vi "AttackerPenalty.vi"(4 "AI Parameters":T8={"GotoKick"={"Dist do cone a frente"=150.0, "attacker farback"=1500.0, "Perto"=300.0, "min dist to kick"=150.0, "kick eps"=0.0, "Time to transition"=0.05}, "Attacker"={"CC chute"=0.09, "CC passe"=0.045, "Kick Force"=100.0, "ball-robot Kick"=200.0, "ball-robot Pass"=0.3, "drible\nAttk"=FALSE}, "Defender"={"D max"=1700.0, "Vel p/ robô av"=1000.0, "Kick Force"=100.0, "D atk-def"=0.0, "D farback"=0.0, "drible\ndef"=FALSE, "drible\ngoalie"=FALSE}, "Timeout"={"Field/v in x"=6.0, "Dist Robots"=300, "Dist up in y"=300}, "Pose Striker"={"dist"=200.0, "Numeric"=-4.0, "dist 2"=200.0, "drible\nstriker"=FALSE}, "Dist Stop"=300.0, "D ball out"=200, "D central gap "=150.0, "T pass"=0.0, "Force ++"=0.0, "range kick"=0.0, "Chute alto"=TRUE, "Marcador novo"=TRUE, "drible"=FALSE, "D drible"=300.0, "Versão Striker"=enum."Auto", "Defesa"=enum."ManMark", "Marcador"=enum."Marcar Segundo mais perigoso", "Receptor passe"=enum."Auto", "Área"=enum."Quadrada", "Decisão\nsimples?"=FALSE} {"D drible" format="%#_13g"; "D central gap" format="%#_13g"; "Dist Stop" format="%#_13g"; "Pose Striker"."Numeric" format="%#_13g"; "Defender"."Kick Force" format="%#_13g"; "Defender"."Vel p/ robô av" format="%#_13g"; "Attacker"."ball-robot Kick" format="%#_13g"; "Attacker"."Kick Force" format="%#_13g"; "Attacker"."CC passe" format="%#_13g"; "Attacker"."CC chute" format="%#_13g"; "GotoKick"."kick eps" format="%#_13g"; "GotoKick"."min dist to kick" format="%#_13g"; "GotoKick"."Perto" format="%#_13g"; "GotoKick"."attacker farback" format="%#_13g"; "GotoKick"."Dist do cone a frente" format="%#_13g"}, 7 "IA State Input":T9={"our_robots"=[], "enemy_robots"=[], "balls"=[], "geometry"={"line_width"=0, "field_length"=0, "field_width"=0, "boundary_width"=0, "referee_width"=0, "goal_width"=0, "goal_depth"=0, "goal_wall_width"=0, "center_circle_radius"=0, "defense_radius"=0, "defense_stretch"=0, "free_kick_from_defense_dist"=0, "penalty_spot_from_field_line_dist"=0, "penalty_line_from_spot_dist"=0}, "IA Judge"={"stage"="", "command"="", "our_goalie_id"=0.0, "enemy_goalie_id"=0.0, "command enum"=enum."Halt", "Time"=enum."Azul"}, "Received Timestamp"=timestamp(0 s since 1904-01-01), "Events"={"Touch"=FALSE, "Ball out"=FALSE, "id touch"=0.0, "Ball out of \nVision"=FALSE, "Ball inside \nGoalie area"=FALSE, "Robot not responding"=FALSE, "Robots responding status"=[1.0, 1.0, 1.0, 1.0, 1.0, 1.0], "Enemy Ball \nPossession"=FALSE, "Pass State"=FALSE, "id end of pass"=0.0, "Kick"=FALSE, "Id ini Possession"=0.0, "Ball Possesion"=FALSE, "Id Possesion"=0.0, "Direct Kick"=FALSE, "2nd Strk Ativo"=FALSE}}, 8 "atacando contra?":bool=TRUE, 9 "balls":T6[](array[typedef]), 10 "geometry":T7, 11 "Robot in":T1={"id"=0, "function"=enum."Attacker", "x"=0.0, "y"=0.0, "orientation"=0.0, "v_tangent"=0.0, "v_normal"=0.0, "v_ang"=0.0, "kick_x"=0.0, "kick_z"=0.0, "dribble"=FALSE, "Timestamp"=timestamp(0 s since 1904-01-01), "estimatives"={"est_v_tangent"=0.0, "est_v_normal"=0.0, "est_vx"=0.0, "est_vy"=0.0, "Pos Robot Est"=[]}, "dest_x_kick"=0.0, "dest_y_kick"=0.0, "Gap Coord"=[], "States"=enum."GoToTangent", "Path "=[], "Path  Smooth"=[], "Dest"=[]}) -> (2 "Robot out":T1={"id"=5, "function"=enum."Attacker", "x"=-1842.5054931640625, "y"=520.60986328125, "orientation"=-2.7555055618286133, "v_tangent"=-0.08361641967936218, "v_normal"=-0.20513016702014014, "v_ang"=0.24456003022714357, "kick_x"=0.0, "kick_z"=0.0, "dribble"=FALSE, "Timestamp"=timestamp(2082758857.4639893 s since 1904-01-01), "estimatives"={"est_v_tangent"=0.0, "est_v_normal"=0.0, "est_vx"=0.0, "est_vy"=0.0, "Pos Robot Est"=[]}, "dest_x_kick"=0.0, "dest_y_kick"=0.0, "Gap Coord"=[], "States"=enum."GoToTangent", "Path "=[], "Path  Smooth"=[], "Dest"=[]})   [LabVIEW 2018]
uses:
  Core/AI Input.ctl
  Core/AI Robot.ctl
  Functions Enum.ctl
  AttackerStates.ctl
  Path Planning/RRT/PathDests.ctl
  Path Planning/RRT/PathDest.ctl
  Core/AI Ball.ctl
  Core/Field Size.ctl
  Core/AI Judge.ctl
  Command Enum.ctl
  Util/Events/Events.ctl
  AI Parameters.ctl
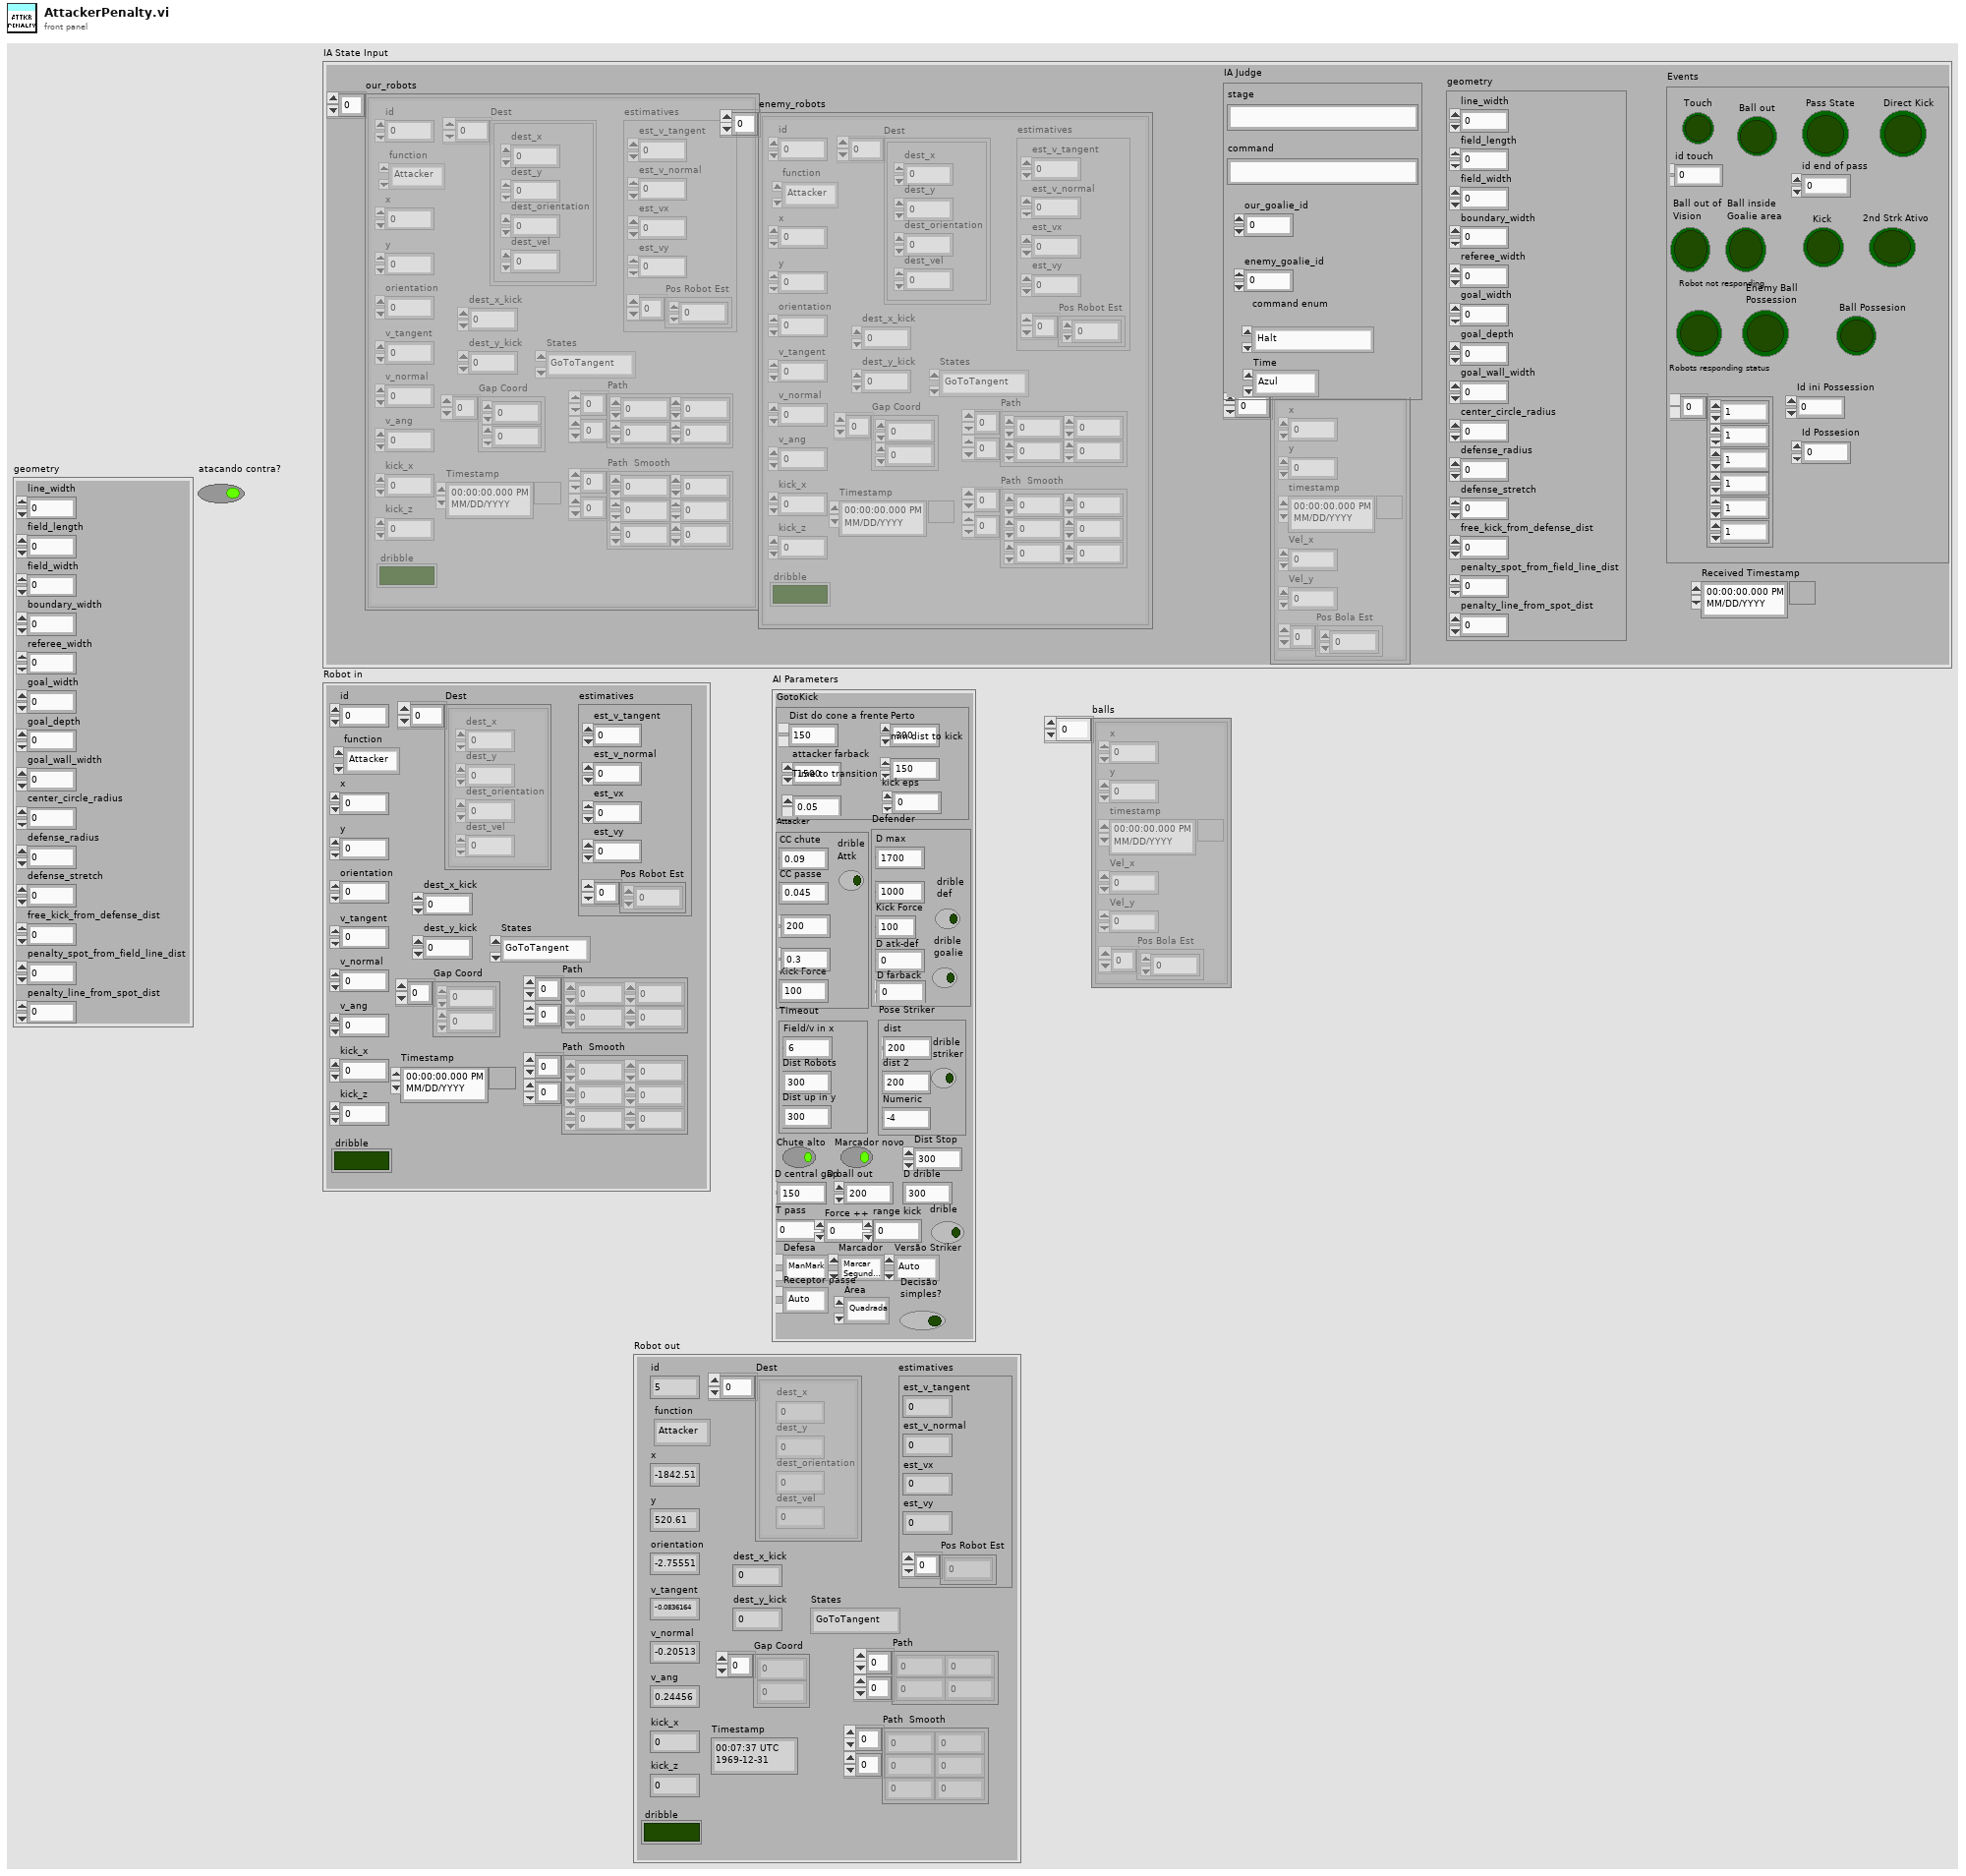
[diagram p1: front panel]
types:
  T1 = typedef "AI Robot.ctl" = cluster{"id":u32, "function":T2, "x":dbl, "y":dbl, "orientation":dbl, "v_tangent":dbl, "v_normal":dbl, "v_ang":dbl, "kick_x":dbl, "kick_z":dbl, "dribble":bool, "Timestamp":timestamp, "estimatives":cluster{"est_v_tangent":dbl, "est_v_normal":dbl, "est_vx":dbl, "est_vy":dbl, "Pos Robot Est":dbl[]}, "dest_x_kick":dbl, "dest_y_kick":dbl, "Gap Coord":dbl[], "States":T3, "Path ":dbl[][], "Path  Smooth":dbl[][], "Dest":T4}
  T2 = typedef "Functions Enum.ctl" = enum16{"2nd Striker", "Attacker", "Goalie", "Defender", "Striker", "Goto 0", "Dummy", "Kicker", "ZigZag 0", "ZigZag 1", "ZigZag 2", "ZigZag 3", "ZigZag 4", "ZigZag 5", "ZigZag 6", "ZigZag 7", "ZigZag 8", ""}
  T3 = typedef "AttackerStates.ctl" = enum16{"Pass", "GoToTangent", "BallGetting", "GoToKick", ""}
  T4 = typedef "PathDests.ctl" = T5[]
  T5 = typedef "PathDest.ctl" = cluster{"dest_x":dbl, "dest_y":dbl, "dest_orientation":dbl, "dest_vel":dbl}
  T6 = typedef "AI Ball.ctl" = cluster{"x":dbl, "y":dbl, "timestamp":timestamp, "Vel_x":dbl, "Vel_y":dbl, "Pos Bola Est":dbl[]}
  T7 = typedef "Field Size.ctl" = cluster{"line_width":u32, "field_length":u32, "field_width":u32, "boundary_width":u32, "referee_width":u32, "goal_width":u32, "goal_depth":u32, "goal_wall_width":u32, "center_circle_radius":u32, "defense_radius":u32, "defense_stretch":u32, "free_kick_from_defense_dist":u32, "penalty_spot_from_field_line_dist":u32, "penalty_line_from_spot_dist":u32}
  T8 = typedef "AI Parameters.ctl" = cluster{"GotoKick":cluster{"Dist do cone a frente":dbl, "attacker farback":dbl, "Perto":dbl, "min dist to kick":dbl, "kick eps":dbl, "Time to transition":dbl}, "Attacker":cluster{"CC chute":dbl, "CC passe":dbl, "Kick Force":dbl, "ball-robot Kick":dbl, "ball-robot Pass":dbl, "drible\nAttk":bool}, "Defender":cluster{"D max":dbl, "Vel p/ robô av":dbl, "Kick Force":dbl, "D atk-def":dbl, "D farback":dbl, "drible\ndef":bool, "drible\ngoalie":bool}, "Timeout":cluster{"Field/v in x":dbl, "Dist Robots":u32, "Dist up in y":u32}, "Pose Striker":cluster{"dist":dbl, "Numeric":dbl, "dist 2":dbl, "drible\nstriker":bool}, "Dist Stop":dbl, "D ball out":i32, "D central gap ":dbl, "T pass":dbl, "Force ++":dbl, "range kick":dbl, "Chute alto":bool, "Marcador novo":bool, "drible":bool, "D drible":dbl, "Versão Striker":enum16{"Auto", "3", "2", "1"}, "Defesa":enum16{"ManMark", "Barreira"}, "Marcador":enum16{"Marcar Segundo mais perigoso", "Marcar o mais perigoso"}, "Receptor passe":enum16{"Auto", "2nd Striker", "Striker"}, "Área":enum16{"Quadrada", "Circular"}, "Decisão\nsimples?":bool}
  T9 = typedef "AI Input.ctl" = cluster{"our_robots":T1[], "enemy_robots":T1[], "balls":T6[], "geometry":T7, "IA Judge":T10, "Received Timestamp":timestamp, "Events":T12}
  T10 = typedef "AI Judge.ctl" = cluster{"stage":string, "command":string, "our_goalie_id":dbl, "enemy_goalie_id":dbl, "command enum":T11, "Time":enum16{"Azul", "Amarelo"}}
  T11 = typedef "Command Enum.ctl" = enum16{"Halt", "Stop", "Force Start", "PKA Normal Start", "Prepare Kickoff Ally", "PKE Normal Start", "Prepare Kickoff Enemy", "Prepare Penalty Ally", "PPA Normal Start", "Prepare Penalty Enemy", "PPE Normal Start", "Direct Free Enemy", "Direct Free Ally", "Indirect Free Enemy", "Indirect Free Ally", "Timeout Enemy", "Timeout Ally", "Goal Enemy", "Goal Ally", "Ball Placement Enemy", "Ball Placement Ally", "Normal Half Time", "Extra Time Break", "Extra Half Time", "None", "Post Game"}
  T12 = typedef "Events.ctl" = cluster{"Touch":bool, "Ball out":bool, "id touch":dbl, "Ball out of \nVision":bool, "Ball inside \nGoalie area":bool, "Robot not responding":bool, "Robots responding status":dbl[], "Enemy Ball \nPossession":bool, "Pass State":bool, "id end of pass":dbl, "Kick":bool, "Id ini Possession":dbl, "Ball Possesion":bool, "Id Possesion":dbl, "Direct Kick":bool, "2nd Strk Ativo":bool}
  T13 = cluster{"CC chute":dbl, "CC passe":dbl, "Kick Force":dbl, "ball-robot Kick":dbl, "ball-robot Pass":dbl, "drible\nAttk":bool}
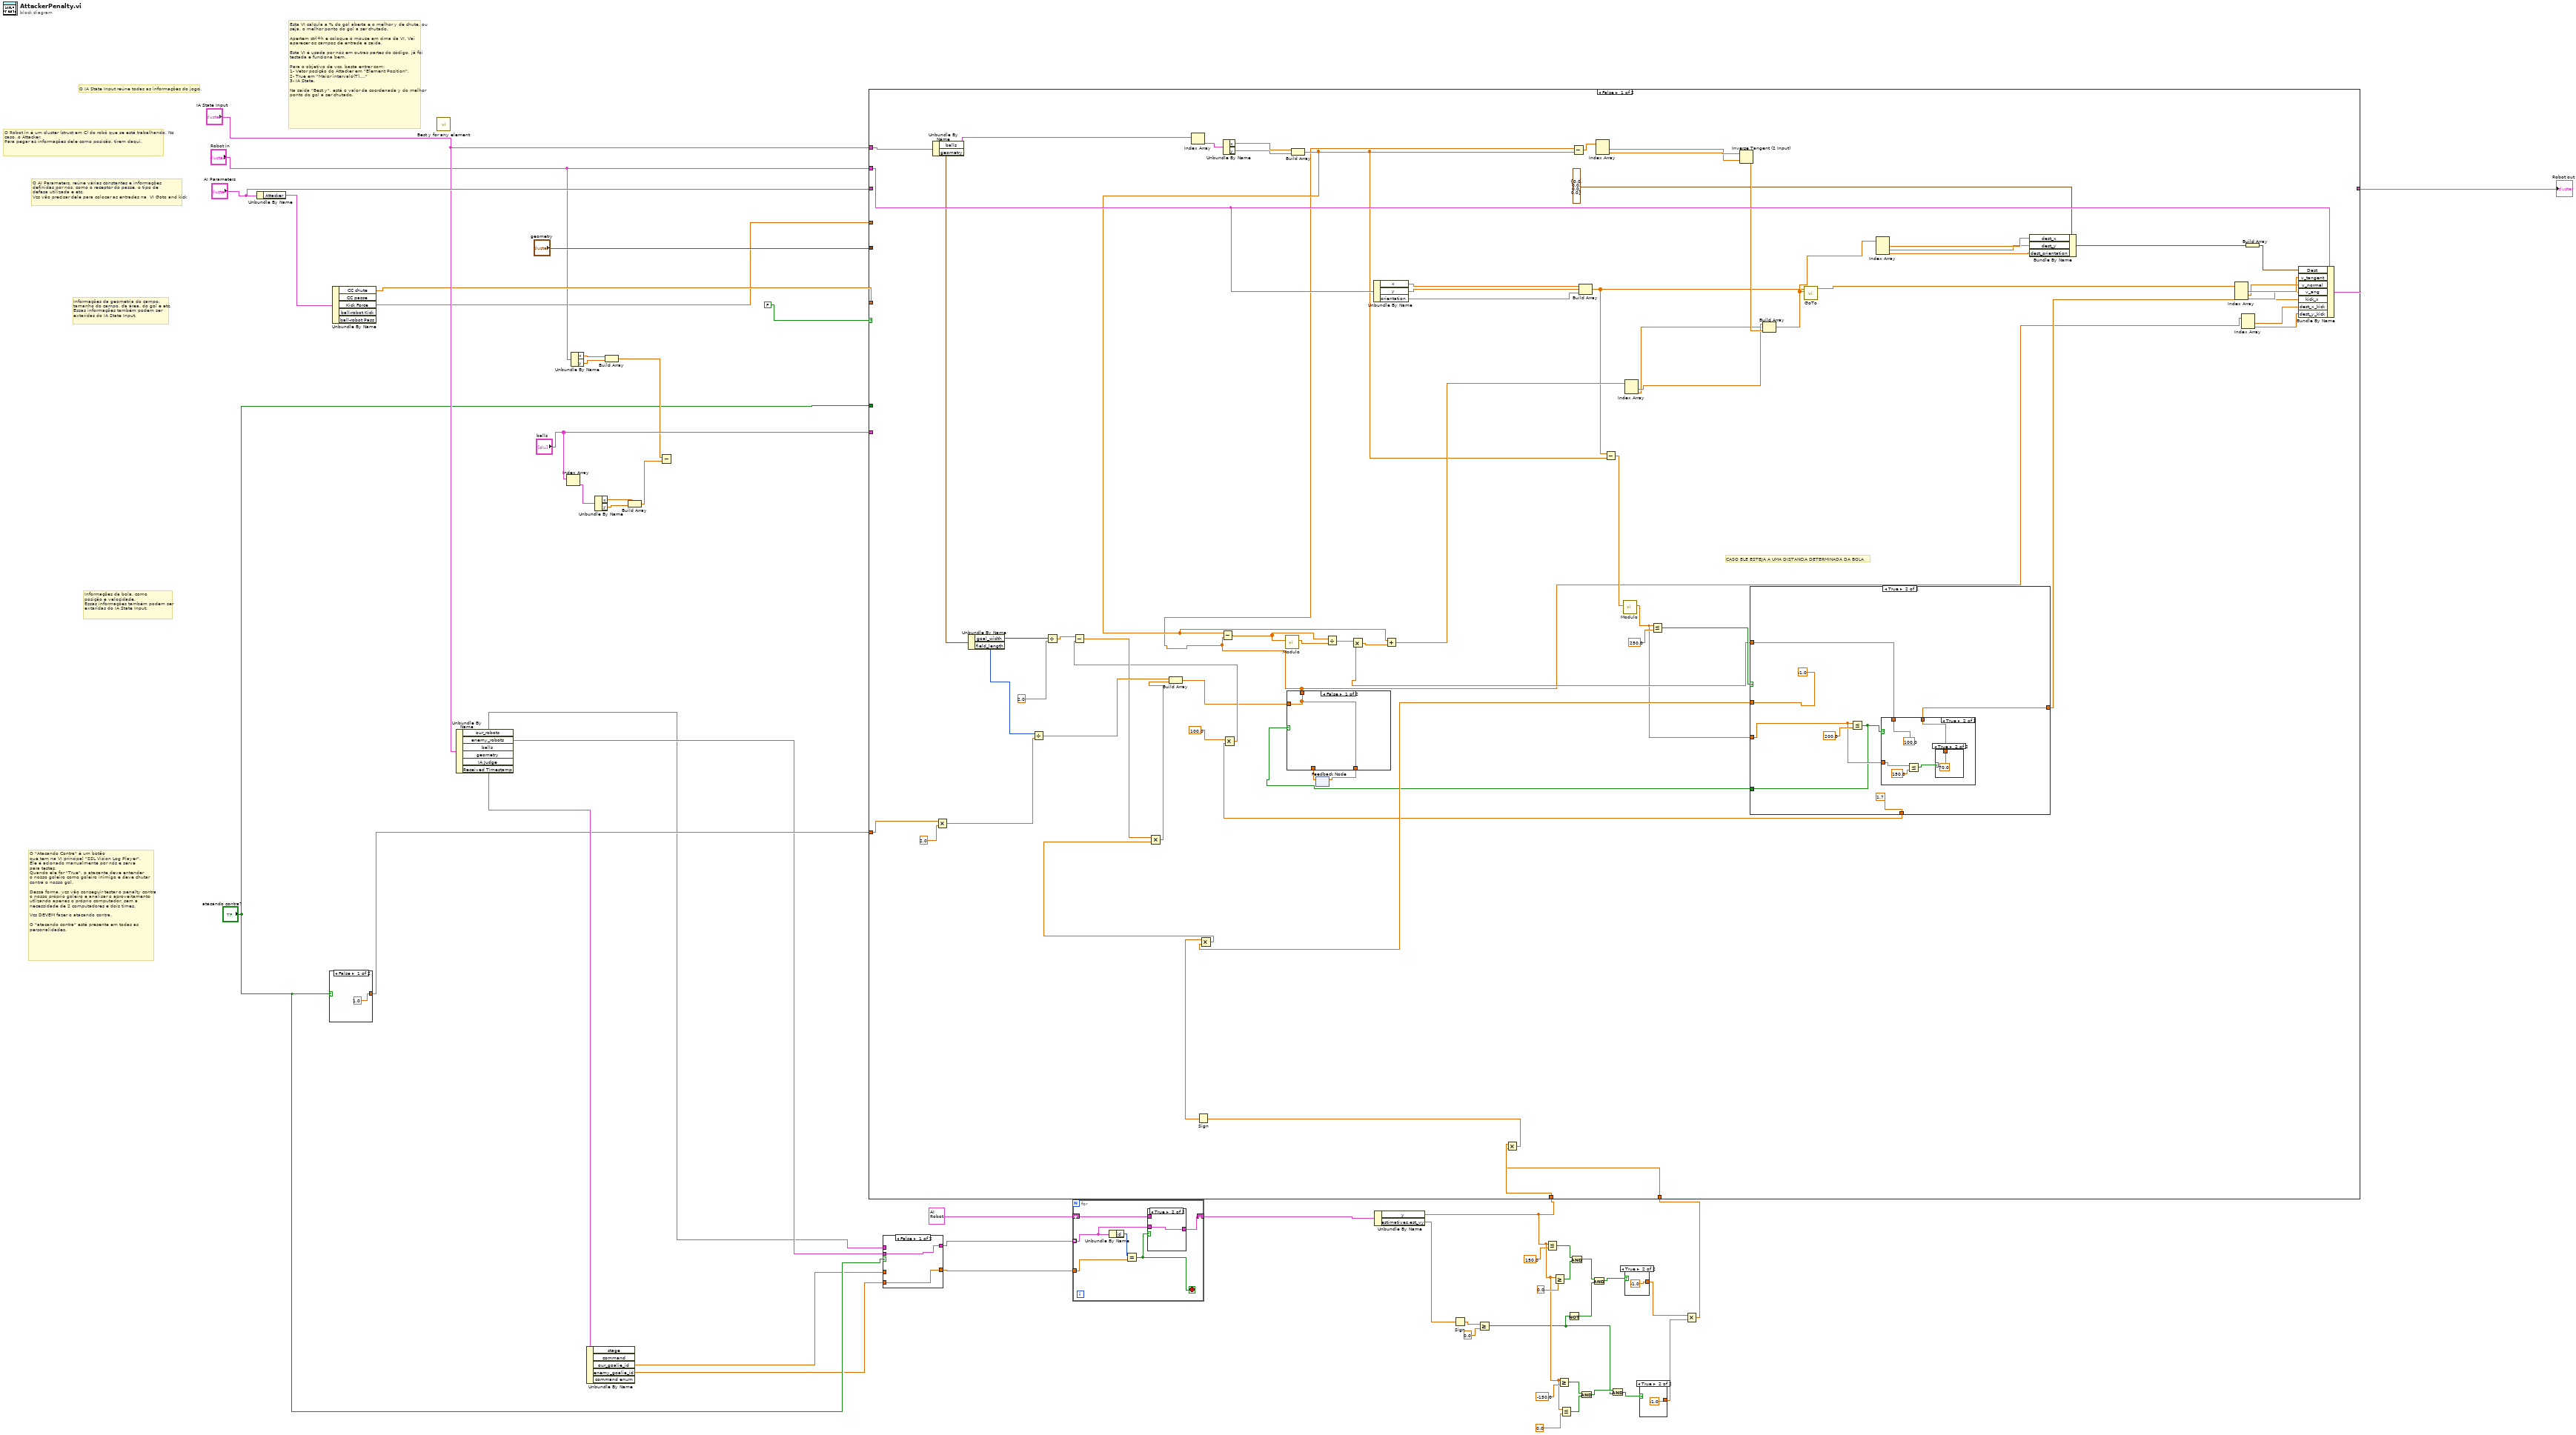
[diagram p0: block diagram]
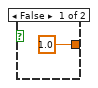
[diagram p2: hidden frame]
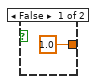
[diagram p3: hidden frame]
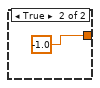
[diagram p5: hidden frame]
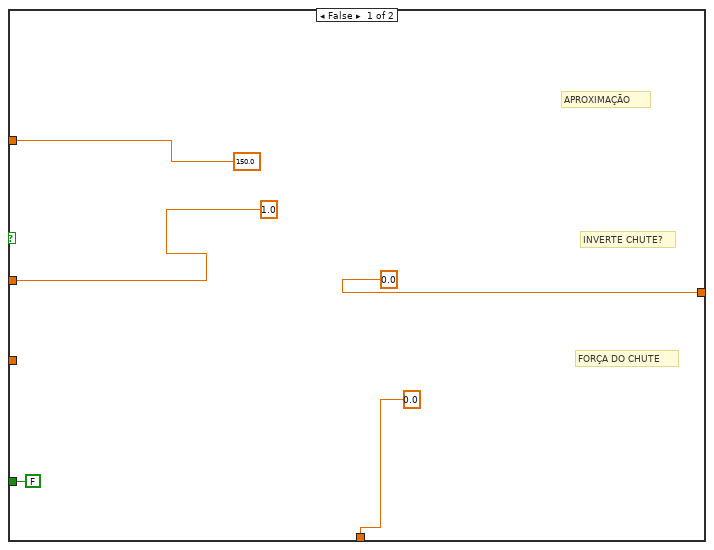
[diagram p8: hidden frame]
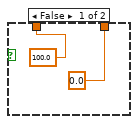
[diagram p9: hidden frame]
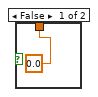
[diagram p10: hidden frame]
diagram:
  # "O \"Atacando Contra\" é um botão\nque tem na VI principal \"SSL Vision Log Player\".\nEle é acionado manualmente por nós e serve\npara testes.\nQuando ele for \"True\", o atacante deve entender \no nosso goleiro como goleiro inimigo e deve chutar\ncontra o nosso gol.\n\nDessa forma, vcs vão conseguir testar o penalty contra\no nosso próprio goleiro e analisar o aproveitamento\nutlizando apenas o próprio computador, sem a\nnecessidade de 2 computadores e dois times.\n\nVcs DEVEM fazer o atacando contra. \n\nO \"atacando contra\" está presente em todas as\npersonalidades."
  # "Informações da bola, como\nposição e velocidade.\nEssas informações também podem ser\nextarídas do IA State Input."
  # "Informações da geometria do campo.\ntamanho do campo, da área, do gol e etc.\nEssas informações também podem ser\nextarídas do IA State Input."
  # "O AI Parameters, reúne várias constantes e informações\ndefinidas por nós, como o receptor do passe, o tipo de\ndefesa utilizada e etc.\nVcs vão precisar dele para colocar as entradas na  VI Goto and kick"
  # "O Robot in é um cluster (struct em C) do robô que se está trabalhando. No caso, o Attacker.\nPara pegar as informações dele como posicão, tirem daqui."
  # "O IA State Input reúne todas as informações do jogo."
  # "Esta VI calcula a % do gol aberta e o melhor y de chute, ou seja, o melhor ponto do gol a ser chutado.\n\nApertem ctrl+h e coloque o mouse em cima da VI. Vai aparecer os campos de entrada e saída.\n\nEsta VI é usada por nós em outras partes do código, já foi testada e funciona bem.\n\nPara o objetivo de vcs, basta entrar com:\n1- Vetor posição do Attacker em \"Element Position\".\n2- True em \"Maior intervalo(T)....\"\n3- IA State.\n\nNa saída \"Best y\", está o valor da coordenada y do melhor ponto do gol a ser chutado."
  n1 = Unbundle By Name("AI Parameters") -> ("Attacker"=w49:T13)
  n2 = case shown="False" "atacando contra?" {
    tunnel: [1.0 -1.0] -> w44
    frame False {
    }
    frame True {
    }
  }
  n3 = Unbundle By Name(w49) -> ("CC chute"=w42:dbl, "Kick Force"=w23:dbl)  [unwired: 3 out]
  n4 = call "Best y for any element.vi"() -> ()  [unwired: 7 in, 5 out]
  n5 = Unbundle By Name("IA State Input") -> ("our_robots"=w25:T1[], "enemy_robots"=w29:T1[], "IA Judge"=w45:T10)  [unwired: 3 out]
  n6 = Index Array(array="balls") -> (element=w39:T6)  [unwired: 1 in]
  n7 = Unbundle By Name("Robot in") -> ("x"=w36:dbl, "y"=w35:dbl)
  n8 = Unbundle By Name(w45) -> ("our_goalie_id"=w26:dbl, "enemy_goalie_id"=w27:dbl)  [unwired: 3 out]
  n9 = Unbundle By Name(w39) -> ("x"=w40:dbl, "y"=w41:dbl)
  n10 = Build Array(w36, w35) -> (w33:dbl[])
  n11 = Build Array(w40, w41) -> (w34:dbl[])
  n12 = Subtract(x=w33, y=w34) -> ()  [unwired: 1 out]
  n13 = case shown="False" "atacando contra?" {
    tunnel: [w53 w54] -> w30
    tunnel: w29 -> [w53 _]
    tunnel: [w52 w55] -> w28
    tunnel: w27 -> [w52 _]
    tunnel: w26 -> [_ w55]
    tunnel: w25 -> [_ w54]
    frame False {
    }
    frame True {
    }
  }
  n14 = for {
    tunnel: w30 -> [w57] mode=indexing
    tunnel: w28 -> [w61]
    shift-right: [w58] -> w24
    shift-left: T1 {"id"=0, "function"=enum."Attacker", "x"=0.0, "y"=0.0, "orientation"=0.0, "v_tangent"=0.0, "v_normal"=0.0, "v_ang"=0.0, "kick_x"=0.0, "kick_z"=0.0, "dribble"=FALSE, "Timestamp"=timestamp(0 s since 1904-01-01), "estimatives"={"est_v_tangent"=0.0, "est_v_normal"=0.0, "est_vx"=0.0, "est_vy"=0.0, "Pos Robot Est"=[]}, "dest_x_kick"=0.0, "dest_y_kick"=0.0, "Gap Coord"=[], "States"=enum."GoToTangent", "Path "=[], "Path  Smooth"=[], "Dest"=[]} ("Robot") -> [w56]
    stop <- w59 stop-if-true
    n15 = Unbundle By Name(w57) -> ("id"=w60:u32)
    n16 = Equal?(x=w60, y=w61) -> (x = y?=w59:bool)
    n17 = case shown="True" w59 {
      tunnel: [w62 w63] -> w58
      tunnel: w57 -> [_ w63]
      tunnel: w56 -> [w62 _]
      frame False {
      }
      frame True {
      }
    }
  }
  n18 = Unbundle By Name(w24) -> ("y"=w15:dbl, "estimatives.est_vy"=w12:dbl)
  n19 = Sign(1:w12) -> (0:w11:dbl)
  n20 = Greater Or Equal?(x=w11, y=0.0) -> (x >= y?=w7:bool)
  n21 = Less Or Equal?(x=w15, y=150.0) -> (x <= y?=w20:bool)
  n22 = Greater Or Equal?(x=w15, y=0.0) -> (x >= y?=w18:bool)
  n23 = Greater Or Equal?(x=w15, y=-150.0) -> (x >= y?=w14:bool)
  n24 = Less Or Equal?(x=w15, y=0.0) -> (x <= y?=w13:bool)
  n25 = Not(x=w7) -> (.not. x?=w6:bool)
  n26 = And(x=w20, y=w18) -> (x .and. y?=w9:bool)
  n27 = And(x=w14, y=w13) -> (x .and. y?=w8:bool)
  n28 = And(x=w9, y=w6) -> (x .and. y?=w4:bool)
  n29 = And(x=w8, y=w7) -> (x .and. y?=w5:bool)
  n30 = case shown="True" w4 {
    tunnel: [1.0 -1.0] -> w3
    frame False {
    }
    frame True {
    }
  }
  n31 = case shown="True" w5 {
    tunnel: [1.0 -1.0] -> w2
    frame False {
    }
    frame True {
    }
  }
  n32 = Multiply(x=w3, y=w2) -> (x*y=w1:dbl)
  n33 = case shown="False" FALSE {
    tunnel: [w134 w158] -> w48
    tunnel: "AI Parameters" -> [_ _]
    tunnel: "IA State Input" -> [w127 _]
    tunnel: "Robot in" -> [w130 w158]
    tunnel: w44 -> [w95 _]
    tunnel: "atacando contra?" -> [_ _]
    tunnel: "geometry" -> [_ _]
    tunnel: "balls" -> [_ _]
    tunnel: w42 -> [_ _]
    tunnel: w23 -> [_ _]
    tunnel: w15 -> [w70 _]
    tunnel: w1 -> [w68 _]
    frame False {
      # "CASO ELE ESTEJA A UMA DISTANCIA DETERMINADA DA BOLA"
      n34 = Unbundle By Name(w127) -> ("balls"=w110:T6[], "geometry"=w119:T7)
      n35 = Multiply(x=w95, y=2.0) -> (x*y=w93:dbl)
      n36 = Unbundle By Name(w119) -> ("goal_width"=w108:u32, "field_length"=w105:u32)
      n37 = Divide(x=w105, y=w93) -> (x/y=w104:dbl)
      n38 = Divide(x=w108, y=2.0) -> (x/y=w106:dbl)
      n39 = Index Array(array=w110) -> (element=w126:T6)  [unwired: 1 in]
      n40 = Unbundle By Name(w126) -> ("x"=w125:dbl, "y"=w124:dbl)
      n41 = Build Array(w125, w124) -> (w74:dbl[])
      n42 = feedback #1() -> (w76:dbl[])  [unwired: 1 in]
      n43 = Unbundle By Name(w130) -> ("x"=w111:dbl, "y"=w129:dbl, "orientation"=w128:dbl)
      n44 = Multiply(x=w70, y=w68) -> (x*y=w69:dbl)
      n45 = Sign(1:w69) -> (0:w86:dbl)
      n46 = Build Array(w111, w129, w128) -> (w92:dbl[])
      n47 = Subtract(x=w92, y=w74) -> (x-y=w91:dbl[])
      n48 = call "Modulo.vi"("2D vector"=w91) -> ("Modulo"=w83:dbl)  [unwired: 10 in]
      n49 = Less Or Equal?(x=w83, y=250.0) -> (x <= y?=w89:bool)
      n50 = case shown="True" w89 {
        tunnel: [150.0 w145] -> w88
        tunnel: [1.0 -1.0] -> w85
        tunnel: [0.0 w147] -> w84
        tunnel: w83 -> [_ w143]
        tunnel: [0.0 1.7] -> w80
        tunnel: [FALSE w142] -> w75
        frame False {
          # "FORÇA DO CHUTE"
          # "INVERTE CHUTE?"
          # "APROXIMAÇÃO"
        }
        frame True {
          n51 = Less Or Equal?(x=w143, y=200.0) -> (x <= y?=w142:bool)
          n52 = case shown="True" w142 {
            tunnel: [0.0 w151] -> w147
            tunnel: [100.0 100.0] -> w145
            tunnel: w143 -> [_ w154]
            frame False {
            }
            frame True {
              n53 = Less Or Equal?(x=w154, y=150.0) -> (x <= y?=w152:bool)
              n54 = case shown="True" w152 {
                tunnel: [0.0 70.0] -> w151
                frame False {
                }
                frame True {
                }
              }
            }
          }
        }
      }
      n55 = Multiply(x=w86, y=w85) -> (x*y=w87:dbl)
      n56 = Multiply(x=100.0, y=w80) -> (x*y=w82:dbl)
      n57 = Subtract(x=w106, y=w82) -> (x-y=w103:dbl)
      n58 = Multiply(x=w103, y=w87) -> (x*y=w102:dbl)
      n59 = Build Array(w104, w102) -> (w73:dbl[])
      n60 = case shown="False" w75 {
        tunnel: [w135 w136] -> w71
        tunnel: w73 -> [w135 _]
        tunnel: [w135 w136] -> w77
        tunnel: w76 -> [_ w136]
        frame False {
        }
        frame True {
        }
      }
      n61 = Subtract(x=w74, y=w71) -> (x-y=w72:dbl[])
      n62 = call "Modulo.vi"("2D vector"=w72) -> ("Modulo"=w101:dbl)  [unwired: 10 in]
      n63 = feedback-in #1(w77) -> ()
      n64 = Divide(x=w72, y=w101) -> (x/y=w100:dbl[])
      n65 = Multiply(x=w100, y=w88) -> (x*y=w99:dbl[])
      n66 = Add(x=w74, y=w99) -> (x+y=w98:dbl[])
      n67 = Subtract(x=w71, y=w74) -> (x-y=w123:dbl[])
      n68 = Index Array(array=w123) -> (element #1=w121:dbl, element #2=w122:dbl)  [unwired: 2 in]
      n69 = Index Array(array=w98) -> (element #1=w97:dbl, element #2=w96:dbl)  [unwired: 2 in]
      n70 = Inverse Tangent (2 Input)(1:w121, 2:w122) -> (0:w120:dbl)
      n71 = Build Array(w97, w96, w120) -> (w113:dbl[])
      n72 = call "GoTo.vi"("Target"=w113, "Position"=w92) -> ("Output\nVelocity"=w133:dbl[])  [unwired: 8 in, 1 out]
      n73 = Index Array(array=w113) -> (element #1=w117:dbl, element #2=w116:dbl, element #3=w115:dbl)  [unwired: 3 in]
      n74 = Bundle By Name(cluster=T5 {"dest_x"=0.0, "dest_y"=0.0, "dest_orientation"=0.0, "dest_vel"=0.0} ("element"), "dest_x"=w117, "dest_y"=w116, "dest_orientation"=w115) -> (w114:T5)
      n75 = Index Array(array=w133) -> (element #1=w132:dbl, element #2=w131:dbl, element #3=w109:dbl)  [unwired: 3 in]
      n76 = Index Array(array=w71) -> (element #1=w79:dbl, element #2=w78:dbl)  [unwired: 2 in]
      n77 = Build Array(w114) -> (w112:T5[])
      n78 = Bundle By Name(cluster=w130, "Dest"=w112, "v_tangent"=w132, "v_normal"=w131, "v_ang"=w109, "kick_x"=w84, "dest_x_kick"=w79, "dest_y_kick"=w78) -> (w134:T1)
    }
    frame True {
    }
  }
  "Robot out" <- w48
